vi "Initialize MeasurementLink Session.vi"(7 "remote connection options":T2, 8 "error in":errorcluster, 9 "initialize and close session behavior":T1, 10 "session initialization parameters":T3, 11 "session factory in":refnum<class "Session Factory.lvclass">) -> (0 "error out":errorcluster, 2 "session out":variant, 3 "session factory out":refnum<class "Session Factory.lvclass">)   [LabVIEW 2021, in "Session Management niDAQmx.lvlib" / "Session Factory.lvclass"]
doc: "Creates a new session using the provided <b>session initialization parameters</b>. If the session represents a remote session, <b>initialize and close session behavior</b> determines whether creating the local session creates a new session on the server or attaches to an existing session on the server."
uses:
  Session Factory.lvclass
  <vilib>/Plug-In SDKs/Sessions/Instrument/ISession Factory/Session Initialization Parameters.ctl
  <vilib>/Plug-In SDKs/Sessions/Instrument/ISession Factory/Remote Connection Options.ctl
  <vilib>/Plug-In SDKs/Sessions/Instrument/ISession Factory/Initialize and Close Session Behavior.ctl
  Client/NI_DAQmx_client/RPC Messages/nidaqmx_grpc_CreateTaskRequest.ctl
  Client/NI_DAQmx_client/RPC Messages/nidevice_grpc_SessionInitializationBehavior.ctl
  Client/NI_DAQmx_client/RPC Messages/nidevice_grpc_Session_session/nidevice_grpc_Session_session.lvclass/nidevice_grpc_Session_session.ctl
  Session Factory.lvclass/Session Factory.ctl
  Client/NI_DAQmx_client/NI_DAQmx_client.lvlib
  Session Management niDAQmx.lvlib
  Client/NI_DAQmx_client/RPC Messages/nidevice_grpc_Session_session/nidevice_grpc_Session_session.lvclass
  <vilib>/Plug-In SDKs/Sessions/Instrument/ISession Factory/ISession Factory.lvclass
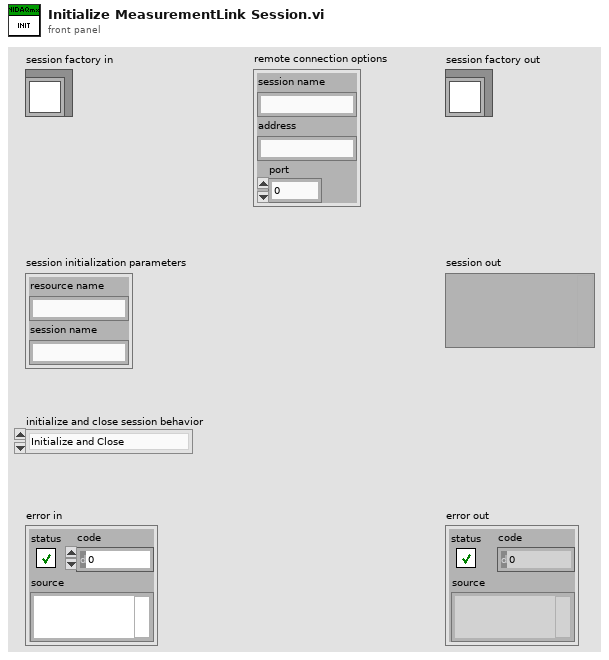
[diagram p1: front panel]
types:
  T1 = typedef "NI Session Management Instrument.lvlib/ISession Factory.lvclass/Initialize and Close Session Behavior.ctl" = enum16{"Initialize and Close", "Attach and Detach", "Initialize and Detach", "Attach and Close"}
  T2 = typedef "NI Session Management Instrument.lvlib/ISession Factory.lvclass/Remote Connection Options.ctl" = cluster{"session name":string, "address":string, "port":u32}
  T3 = typedef "NI Session Management Instrument.lvlib/ISession Factory.lvclass/Session Initialization Parameters.ctl" = cluster{"resource name":string, "session name":string}
  T4 = typedef "NI_DAQmx_client.lvlib/nidaqmx_grpc_CreateTaskRequest.ctl" = cluster{"session_name":string, "initialization_behavior":T5}
  T5 = typedef "NI_DAQmx_client.lvlib/nidevice_grpc_SessionInitializationBehavior.ctl" = enum32{"SESSION_INITIALIZATION_BEHAVIOR_UNSPECIFIED", "SESSION_INITIALIZATION_BEHAVIOR_INITIALIZE_NEW", "SESSION_INITIALIZATION_BEHAVIOR_ATTACH_TO_EXISTING"}
  T6 = typedef "grpc-lvsupport-release.lvlib/grpcId.ctl" = u64
  T7 = typedef "NI_DAQmx_client.lvlib/nidaqmx_grpc_CreateTaskResponse.ctl" = cluster{"status":i32, "task":T8, "new_session_initialized":bool}
  T8 = typedef "NI_DAQmx_client.lvlib/nidevice_grpc_Session.ctl" = cluster{"nidevice_grpc_Session_session":refnum<class "nidevice_grpc_Session_session.lvclass">}
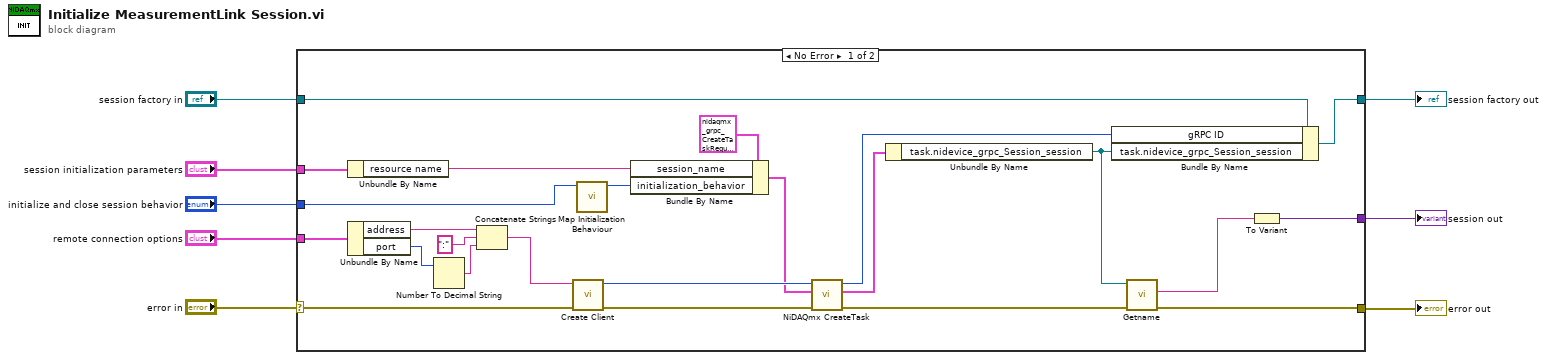
[diagram p0: block diagram]
diagram:
  n1 = case shown="No Error" "error in" {
    selector: "error in" -> [w26 w33]
    tunnel: "session factory in" -> [w16 w34]
    tunnel: [w17 w34] -> w3
    tunnel: "remote connection options" -> [w29 _]
    tunnel: "session initialization parameters" -> [w32 _]
    tunnel: "initialize and close session behavior" -> [w20 _]
    tunnel: [w11 w33] -> w2
    tunnel: [w13 _] -> w1
    frame No Error {
      n2 = Unbundle By Name(w32) -> ("resource name"=w21:string)
      n3 = Unbundle By Name(w29) -> ("address"=w28:string, "port"=w27:u32)
      n4 = Number To Decimal String(number=w27) -> (decimal integer string=w30:string)  [unwired: 1 in]
      n5 = Concatenate Strings(w28, ":" ("string"), w30) -> (w25:string)
      n6 = call "Create Client.vi"("error in"=w26, "address"=w25) -> ("error out"=w24:errorcluster, "gRPC ID Out"=w23:T6)  [unwired: 8 in]
      n7 = call "Map Initialization Behaviour.vi"("initialize and close session behavior in"=w20) -> ("initialization_behavior"=w19:T5)  [unwired: 10 in]
      n8 = Bundle By Name(cluster=T4 {"session_name"="", "initialization_behavior"=enum."SESSION_INITIALIZATION_BEHAVIOR_UNSPECIFIED"} ("Request Data"), "session_name"=w21, "initialization_behavior"=w19) -> (w18:T4)
      n9 = call "NiDAQmx CreateTask.vi"("error in"=w24, "Request Data"=w18, "gRPC ID"=w23) -> ("error out"=w12:errorcluster, "Response Data"=w14:T7, "gRPC ID out"=w15:T6)  [unwired: 6 in]
      n10 = Unbundle By Name(w14) -> ("task.nidevice_grpc_Session_session"=w10:refnum<class "nidevice_grpc_Session_session.lvclass">)
      n11 = Bundle By Name(cluster=w16, "gRPC ID"=w15, "task.nidevice_grpc_Session_session"=w10) -> (w17:refnum<class "Session Factory.lvclass">)
      n12 = call "Getname.vi"("error in (no error)"=w12, "OneOfTemplate in"=w10) -> ("error out"=w11:errorcluster, "Get_Val"=w9:string)  [unwired: 7 in, 1 out]
      n13 = To Variant(anything=w9) -> (Variant=w13:variant)
    }
    frame Error {
    }
  }
  "error out" <- w2
  "session factory out" <- w3
  "session out" <- w1
